vi "CTR-Initialize.vi"(0 "Config":T1={"enabled"=FALSE, "Hi ticks"=5, "Low ticks"=4995, "Idle state"=10214, "Delay ticks"=0} {"Idle state" items=["High"=10192, "Low"=10214]; "Low ticks" max=1}, 7 "task":refnum<k21>, 11 "error in (no error)":errorcluster) -> (8 "Counter Task":T2={"task"="Counter"}, 15 "error out":errorcluster)   [LabVIEW 2020]
uses:
  Typedefs/CTR-Task Specification.ctl
  Typedefs/CTR-Config.ctl
  <vilib>/DAQmx/create/channels.llb/DAQmx Create Channel (CO-Pulse Generation-Ticks).vi
  <vilib>/DAQmx/configure/timing.llb/DAQmx Timing (Implicit).vi
  <vilib>/DAQmx/configure/trigger.llb/DAQmx Start Trigger (Digital Edge).vi
  <resource>/objmgr/daqmx.rc
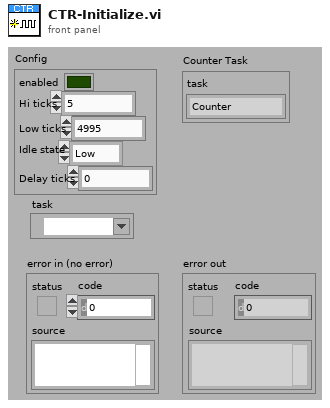
[diagram p1: front panel]
types:
  T1 = typedef "CTR-Config.ctl" = cluster{"enabled":bool, "Hi ticks":u32, "Low ticks":u32, "Idle state":i32, "Delay ticks":u32}
  T2 = typedef "CTR-Task Specification.ctl" = cluster{"task":string}
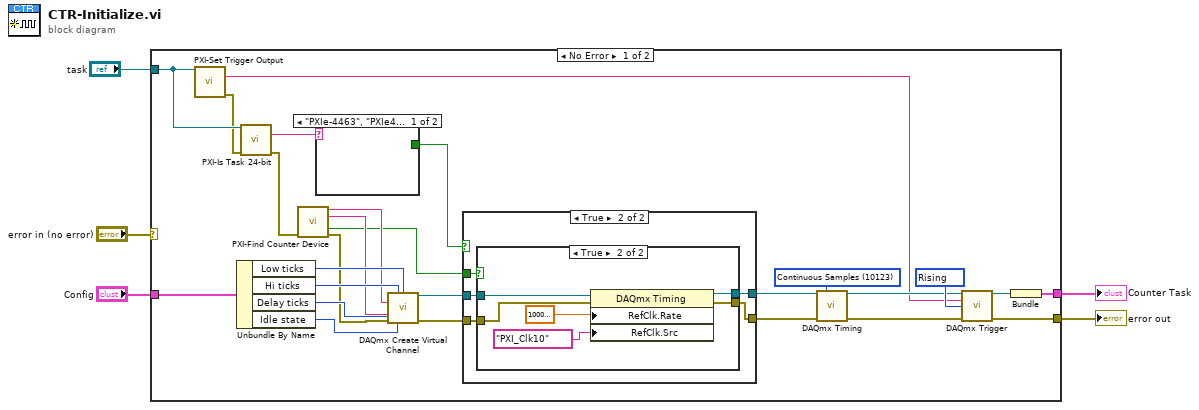
[diagram p0: block diagram]
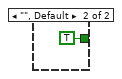
[diagram p2: hidden frame]
diagram:
  n1 = case shown="No Error" "error in (no error)" {
    selector: "error in (no error)" -> [_ w48]
    tunnel: [w31 w48] -> w5
    tunnel: [w11 _] -> w3
    tunnel: "Config" -> [w10 _]
    tunnel: "task" -> [w9 _]
    frame No Error {
      w29 = 10280 items=["Rising"=10280, "Falling"=10171] ("Trigger Edge")
      w30 = 10123 items=["Finite Samples"=10178, "Continuous Samples"=10123] ("sample mode")
      n2 = call "PXI-Set Trigger Output.vi"("Task in"=w9) -> ("Trigger Terminal"=w8:string, "error out"=w7:errorcluster)  [unwired: 12 in, 1 out]
      n3 = Unbundle By Name(w10) -> ("Low ticks"=w22:u32, "Hi ticks"=w21:u32, "Delay ticks"=w20:u32, "Idle state"=w19:i32)
      n4 = call "PXI-Is Task 24-bit.vi"("task"=w9, "error in (no error)"=w7) -> ("Product Type"=w15:string, "error out"=w6:errorcluster)  [unwired: 8 in, 4 out]
      n5 = call "PXI-Find Counter Device.vi"("error in (no error)"=w6) -> ("Counter Channel"=w17:tag, "RefClk.Src"=w16:tag, "Is M-series board"=w13:bool, "error out"=w18:errorcluster)  [unwired: 10 in, 1 out]
      n6 = case shown="\"PXIe-4463\", \"PXIe4-4464\"" w15 {
        tunnel: [_ TRUE] -> w14
        frame "PXIe-4463", "PXIe4-4464" {
        }
        frame "", Default {
        }
      }
      n7 = call-poly <vilib>:"DAQmx Create Virtual Channel.vi"("high ticks"=w21, "low ticks"=w22, "counter"=w17, "source of ticks"=w16, "error in"=w18, "idle state"=w19, "initial delay"=w20) -> ("task out"=w23:refnum<k21>, "error out"=w24:errorcluster)  [unwired: 7 in]
      n8 = case shown="True" w14 {
        tunnel: [w34 w39] -> w28
        tunnel: [w33 w38] -> w27
        tunnel: w24 -> [w33 w37]
        tunnel: w23 -> [w34 w36]
        tunnel: w13 -> [_ w35]
        frame False {
        }
        frame True {
          n9 = case shown="True" w35 {
            tunnel: [w41 w47] -> w39
            tunnel: [w40 w46] -> w38
            tunnel: w37 -> [w40 w45]
            tunnel: w36 -> [w41 w44]
            frame False {
            }
            frame True {
              n10 = property class="DAQmx Timing"(reference=w44, error in=w45, "RefClk.Rate"=10000000.0, "RefClk.Src"=tag "PXI_Clk10") -> (reference out=w47:refnum<k21>, error out=w46:errorcluster)
            }
          }
        }
      }
      n11 = call-poly <vilib>:"DAQmx Timing.vi"("task/channels in"=w28, "sample mode"=w30, "error in"=w27) -> ("task out"=w26:refnum<k21>, "error out"=w25:errorcluster)  [unwired: 11 in]
      n12 = call-poly <vilib>:"DAQmx Trigger.vi"("task/channels in"=w26, "source"=w8, "edge"=w29, "error in"=w25) -> ("task out"=w12:refnum<k21>, "error out"=w31:errorcluster)  [unwired: 10 in]
      n13 = Bundle("task out"=w12) -> (w11:cluster{"task out":refnum<k21>})  [unwired: 1 in]
    }
    frame Error {
    }
  }
  "error out" <- w5
  "Counter Task" <- w3
